vi "Find Aliases and Routing Channels Sections.vi"(8 "error in (no error)":errorcluster, 11 "Routing and Faulting Custom Device Ref in":T1 format="%.0x") -> (0 "error out":errorcluster, 1 "Routing Channels Ref":T1 format="%.0x", 2 "Aliases Ref":T1 format="%.0x", 3 "Routing and Faulting Custom Device Ref out":T1 format="%.0x")   [LabVIEW 2017, in "Routing and Faulting Scripting.lvlib"]
uses:
  Routing and Faulting Scripting.lvlib
  <vilib>/NI Veristand/Custom Device API/Custom Device Item Ref.ctl
  NationalInstruments.VeriStand.SystemDefinitionAPI
  Shared/Constants.vi
  Shared/Routing and Faulting Shared.lvlib
  <vilib>/NI VeriStand/Custom Device API/Custom Device API.lvlib
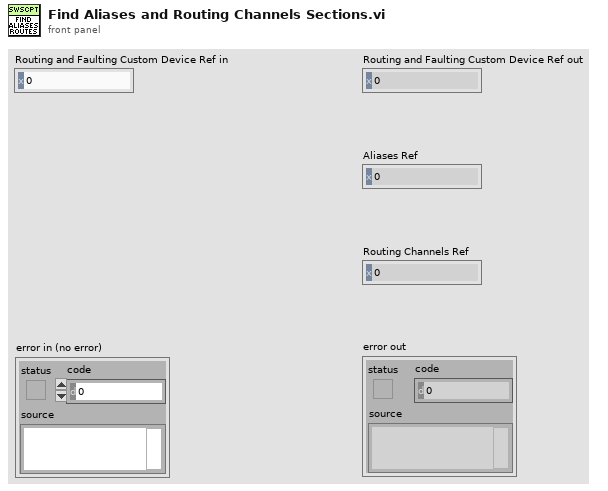
[diagram p1: front panel]
types:
  T1 = typedef "Custom Device API.lvlib/Custom Device Item Ref.ctl" = u64
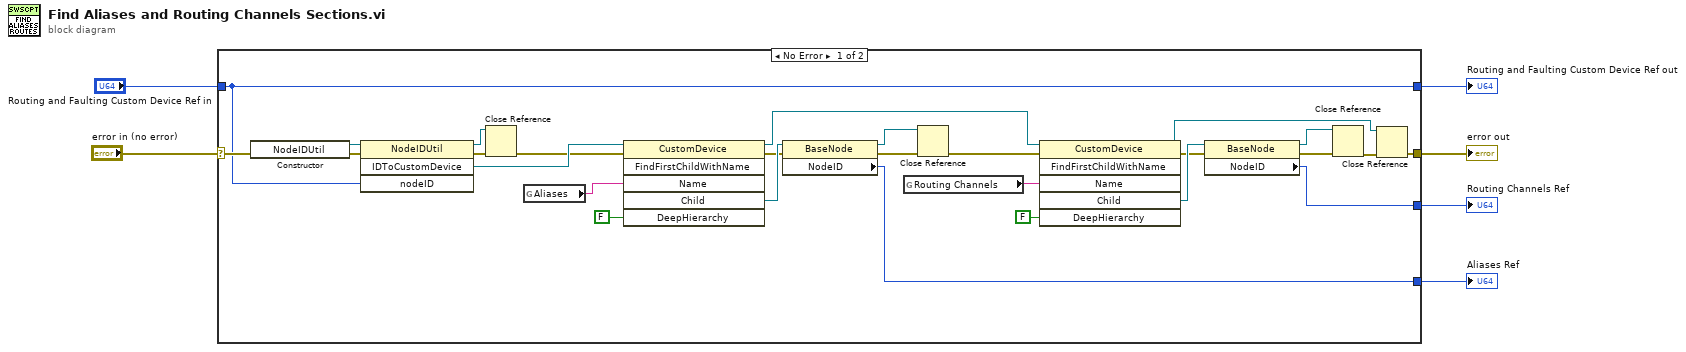
[diagram p0: block diagram]
diagram:
  n1 = case shown="No Error" "error in (no error)" {
    selector: "error in (no error)" -> [w21 w35]
    tunnel: "Routing and Faulting Custom Device Ref in" -> [w10 w34]
    tunnel: [w10 w34] -> w5
    tunnel: [w29 _] -> w4
    tunnel: [w12 w35] -> w3
    tunnel: [w8 _] -> w2
    frame No Error {
      n2 = constructor class="NodeIDUtil"(error in=w21) -> (reference out=w23:refnum<k24>, error out=w24:errorcluster)  [unwired: 2 in, 1 out]
      n3 = invoke class="NodeIDUtil" method="IDToCustomDevice"(reference=w23, error in=w24, "nodeID"=w10) -> (reference out=w19:refnum<k24>, error out=w20:errorcluster, "IDToCustomDevice"=w22:refnum<k24>)  [unwired: 1 in, 1 out]
      n4 = Close Reference(reference=w19, error in (no error)=w20) -> (error out=w18:errorcluster)
      n5 = global read "Constants.vi" "Aliases"() -> (w9:string)
      n6 = invoke class="CustomDevice" method="FindFirstChildWithName"(reference=w22, error in=w18, "Name"=w9, "DeepHierarchy"=FALSE) -> (reference out=w14:refnum<k24>, error out=w31:errorcluster, "Child"=w33:refnum<k24>)  [unwired: 2 in, 3 out]
      n7 = property class="BaseNode"(reference=w33, error in=w31) -> (reference out=w16:refnum<k24>, error out=w17:errorcluster, "NodeID"=w8:u64)
      n8 = global read "Constants.vi" "Routing Channels"() -> (w7:string)
      n9 = Close Reference(reference=w16, error in (no error)=w17) -> (error out=w15:errorcluster)
      n10 = invoke class="CustomDevice" method="FindFirstChildWithName"(reference=w14, error in=w15, "Name"=w7, "DeepHierarchy"=FALSE) -> (reference out=w11:refnum<k24>, error out=w30:errorcluster, "Child"=w32:refnum<k24>)  [unwired: 2 in, 3 out]
      n11 = property class="BaseNode"(reference=w32, error in=w30) -> (reference out=w25:refnum<k24>, error out=w26:errorcluster, "NodeID"=w29:u64)
      n12 = Close Reference(reference=w25, error in (no error)=w26) -> (error out=w13:errorcluster)
      n13 = Close Reference(reference=w11, error in (no error)=w13) -> (error out=w12:errorcluster)
    }
    frame Error {
    }
  }
  "Routing and Faulting Custom Device Ref out" <- w5
  "Aliases Ref" <- w2
  "Routing Channels Ref" <- w4
  "error out" <- w3
